vi "Debouncing Button(SubVI).vi"(9 "millisecond timer value in":u32, 10 "Boolean in":bool, 11 "Land/Take off":bool) -> (2 "millisecond timer value out":u32, 3 "Boolean out":bool)   [LabVIEW 2014]
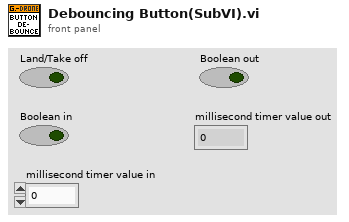
[diagram p1: front panel]
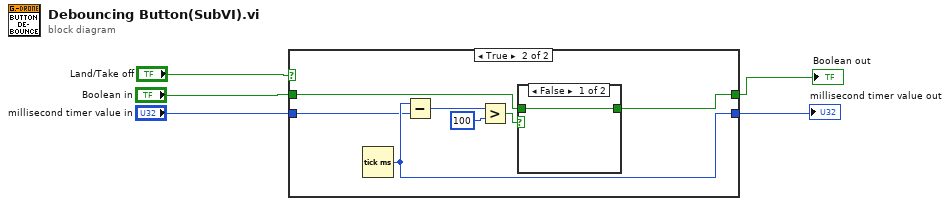
[diagram p0: block diagram]
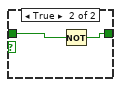
[diagram p3: hidden frame]
diagram:
  n1 = case shown="True" "Land/Take off" {
    tunnel: [w7 w8] -> w1
    tunnel: "Boolean in" -> [w7 w9]
    tunnel: [w6 w14] -> w4
    tunnel: "millisecond timer value in" -> [w6 w13]
    frame False {
    }
    frame True {
      n2 = Tick Count (ms)() -> (millisecond timer value=w14:u32)
      n3 = Subtract(x=w14, y=w13) -> (x-y=w12:u32)
      n4 = Greater?(x=w12, y=u32 100) -> (0:w10:bool)
      n5 = case shown="False" w10 {
        tunnel: w9 -> [w15 w17]
        tunnel: [w15 w16] -> w8
        frame False {
        }
        frame True {
          n6 = Not(x=w17) -> (.not. x?=w16:bool)
        }
      }
    }
  }
  "millisecond timer value out" <- w4
  "Boolean out" <- w1
